vi "FRCts20_WebMethods_ESP_RequestForm.vi"(8 "error in (no error)":errorcluster, 10 "Return Type":T1="mobile", 11 "httpRequestID":u32) -> (0 "error out":errorcluster, 3 "httpRequestID out":u32)   [LabVIEW 2013, in "FRCts20_WebMethods.lvlib"]
uses:
  FRCts20_WebMethods.lvlib
  Backend/source/VI Source/FRCts20_Backend_API/FRCts20_Backend_API.lvlib
  <vilib>/wsapi/NI_WebServices.lvlib
  <vilib>/wsapi/subVIs/Set Integer ESP Variable.vi
  Controls/FRCts20_WebMethods_Globals.vi
  <vilib>/wsapi/subVIs/Set String ESP Variable.vi
  Backend/source/VI Source/INI_Accessor/FRCts20_Backend_INI Controller.lvclass
  Backend/source/VI Source/FRCts20_Backend_API/FRCts20_Backend_API_Event.vi
  Backend/source/VI Source/FRCts20_Backend_API/FRCts20_Backend_API_Event.ctl
  Backend/source/VI Source/FRCts20_Backend_API/FRCts20_Backend_API_Command_Event.ctl
  Backend/source/VI Source/FRCts20_Backend_API/FRCts20_Backend_API_SW.ctl
  Controls/FRCts20_WebMethods_ctl_returntype.ctl
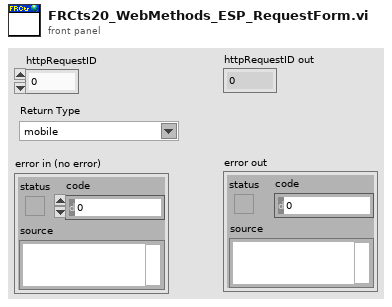
[diagram p1: front panel]
types:
  T1 = typedef "FRCts20_WebMethods.lvlib/FRCts20_WebMethods_ctl_returntype.ctl" = string
  T2 = typedef "FRCts20_Backend_API.lvlib/FRCts20_Backend_API_Command_Event.ctl" = string
  T3 = typedef "FRCts20_Backend_API.lvlib/FRCts20_Backend_API_Event.ctl" = cluster{"Event Index":u32, "Name":string, "Start Time":timestamp, "End Time":timestamp, "Teams":cluster{"Team Index":u32, "Team Number":u32, "Requests":cluster{"Request Number":u32, "Description":string}[], "Has Open Issue":bool}[], "SWType":T4, "APIReturn":string}
  T4 = typedef "FRCts20_Backend_API.lvlib/FRCts20_Backend_API_SW.ctl" = string
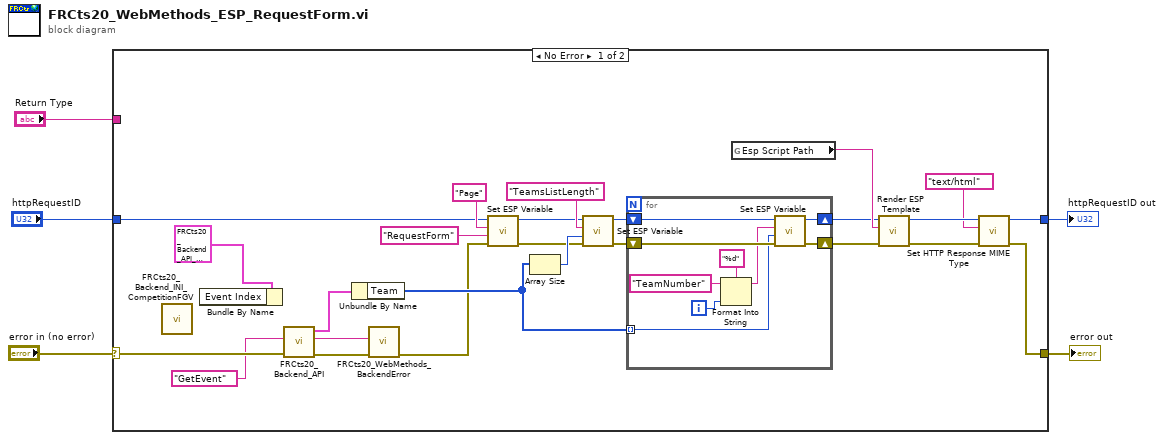
[diagram p0: block diagram]
diagram:
  n1 = case shown="No Error" "error in (no error)" {
    selector: "error in (no error)" -> [w21 w41]
    tunnel: "httpRequestID" -> [w14 w40]
    tunnel: [w20 w40] -> w2
    tunnel: [w19 w41] -> w1
    tunnel: "Return Type" -> [_ _]
    frame No Error {
      n2 = call "FRCts20_Backend_INI_CompetitionFGV.vi"() -> ()  [unwired: 11 in, 1 out]
      n3 = Bundle By Name(cluster=T3 {"Event Index"=0, "Name"="", "Start Time"=timestamp(0 s since 1904-01-01), "End Time"=timestamp(0 s since 1904-01-01), "Teams"=[], "SWType"="", "APIReturn"=""} ("Event In")) -> ()  [unwired: 1 in, 1 out]
      n4 = call-poly "FRCts20_Backend_API.vi"("error in (no error)"=w21, "Command"=T2 "GetEvent") -> ("error out"=w10:errorcluster, "Status"=w9:string, "Event Out"=w30:T3)  [unwired: 7 in]
      n5 = Unbundle By Name(w30) -> ("Team"=w27:u32[])
      n6 = call "FRCts20_WebMethods_BackendError.vi"("error in (no error)"=w10, "Status"=w9) -> ("error out"=w8:errorcluster)  [unwired: 8 in, 1 out]
      n7 = call-poly <vilib>:"Set ESP Variable.vi"("error in (no error)"=w8, "value"="RequestForm", "key"="Page", "httpRequestID"=w14) -> ("error out"=w13:errorcluster, "httpRequestID out"=w15:u32)  [unwired: 6 in]
      n8 = Array Size(array=w27) -> (size(s)=w29:i32)
      n9 = call-poly <vilib>:"Set ESP Variable.vi"("error in (no error)"=w13, "value"=w29, "key"="TeamsListLength", "httpRequestID"=w15) -> ("error out"=w26:errorcluster, "httpRequestID out"=w24:u32)  [unwired: 6 in]
      n10 = for {
        tunnel: w27 -> [w33] mode=indexing
        shift-right: [w38] -> w25
        shift-left: w26 -> [w39]
        shift-right: [w31] -> w11
        shift-left: w24 -> [w37]
        i -> [w35]
        n11 = Format Into String(format string="%d", initial string="TeamNumber", w35) -> (resulting string=w34:string)  [unwired: 1 in, 1 out]
        n12 = call-poly <vilib>:"Set ESP Variable.vi"("error in (no error)"=w39, "value"=w33, "key"=w34, "httpRequestID"=w37) -> ("error out"=w38:errorcluster, "httpRequestID out"=w31:u32)  [unwired: 6 in]
      }
      n13 = global read "FRCts20_WebMethods_Globals.vi" "Esp Script Path"() -> (w18:string)
      n14 = call <vilib>:"Render ESP Template.vi"("error in (no error)"=w25, "espName"=w18, "httpRequestID"=w11) -> ("error out"=w22:errorcluster, "httpRequestID out"=w23:u32)  [unwired: 7 in]
      n15 = call <vilib>:"Set HTTP Response MIME Type.vi"("error in (no error)"=w22, "MIME type (text/html)"="text/html", "httpRequestID"=w23) -> ("error out"=w19:errorcluster, "httpRequestID out"=w20:u32)  [unwired: 7 in]
    }
    frame Error {
    }
  }
  "httpRequestID out" <- w2
  "error out" <- w1
